vi "Preview Pop Up.vi"(6 "Local Data":T1, 7 "UI References":T8, 8 "error in (no error)":errorcluster, 9 "Side":enum16{"Left", "Right"}(ring)=enum."Right", 10 "Coords":T9) -> (0 "error out":errorcluster, 4 "Local Data Out":T1)   [LabVIEW 2024]
uses:
  <vilib>/Utility/miscctls.llb/LVPoint32TypeDef.ctl
  Controls/RVHR - UI Refs.ctl
  Controls/Test Cluster.ctl
  Controls/Excluded Information.ctl
  Controls/Language.ctl
  Controls/Device_Type.ctl
  <vilib>/Utility/miscctls.llb/LVRectTypeDef.ctl
  <vilib>/Utility/miscctls.llb/LVBoundsTypeDef.ctl
  Controls/RVHR - Local Data.ctl
panel:
  out "element":u32
  out "Zoom Picture":picture
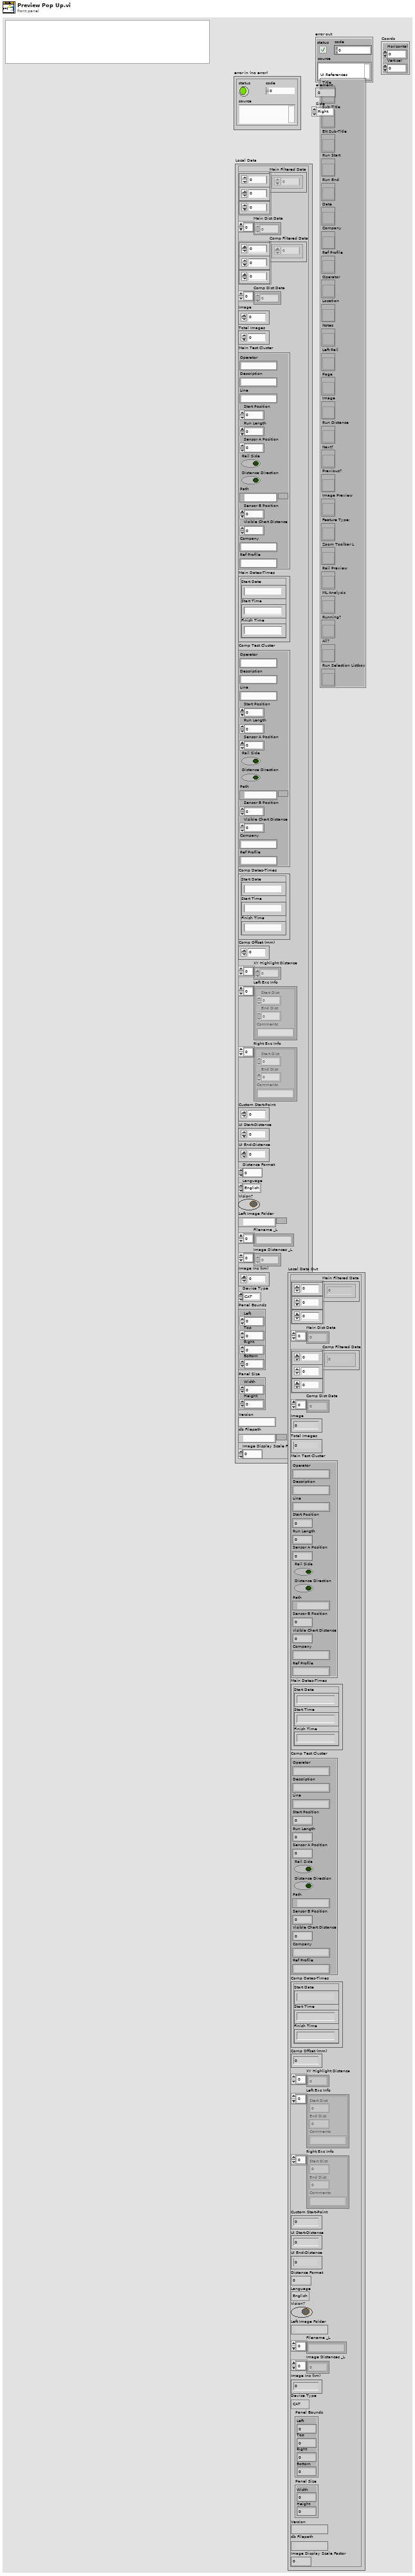
[diagram p1: front panel]
types:
  T1 = typedef "RVHR - Local Data.ctl" = cluster{"Main Filtered Data":dbl[][][], "Main Dist Data":dbl[], "Comp Filtered Data":dbl[][][], "Comp Dist Data":dbl[], "Image":u16, "Total Images":u16, "Main Test Cluster":T2, "Main Dates-Times":cluster{"Start Date":string, "Start Time":string, "Finish Time":string}, "Comp Test Cluster":T2, "Comp Dates-Times":cluster{"Start Date":string, "Start Time":string, "Finish Time":string}, "Comp Offset (mm)":i64, "XY Highlight Distance":dbl[], "Left Exc Info":T3[], "Right Exc Info":T3[], "Custom Start-Point":dbl, "UI Start-Distance":dbl, "UI End-Distance":dbl, "Distance Format":u8, "Language":T4, "Vision?":bool, "Left Image Folder":path, "Filename _L":string[], "Image Distances _L":dbl[], "Image Inc (km)":dbl, "Device Type":T5, "Panel Bounds":T6, "Panel Size":T7, "Version":string, "db Filepath":path, "Image Display Scale Factor":dbl}
  T2 = typedef "Test Cluster.ctl" = cluster{"Operator":string, "Description":string, "Line":string, "Start Position":dbl, "Run Length":dbl, "Sensor A Position":dbl, "Rail Side":bool, "Distance Direction":bool, "Path":path, "Sensor B Position":dbl, "Visible Chart Distance":dbl, "Company":string, "Ref Profile":string}
  T3 = typedef "Excluded Information.ctl" = cluster{"Start Dist":dbl, "End Dist":dbl, "Comments":string}
  T4 = typedef "Language.ctl" = enum16{"English", "Chinese", "German"}
  T5 = typedef "Device_Type.ctl" = enum16{"CAT", "Bi-CAT", "YRCA", "RCA", "RV-HR", "TV-HR"}
  T6 = typedef "LVRectTypeDef.ctl" = cluster{"Left":i16, "Top":i16, "Right":i16, "Bottom":i16}
  T7 = typedef "LVBoundsTypeDef.ctl" = cluster{"Width":u32, "Height":u32}
  T8 = typedef "RVHR - UI Refs.ctl" = cluster{"Title":refnum<vi>, "Sub-Title":refnum<vi>, "EN Sub-Title":refnum<vi>, "Run Start":refnum<vi>, "Run End":refnum<vi>, "Date":refnum<vi>, "Company":refnum<vi>, "Ref Profile":refnum<vi>, "Operator":refnum<vi>, "Location":refnum<vi>, "Notes":refnum<vi>, "Left Rail":refnum<vi>, "Page":refnum<vi>, "Image":refnum<vi>, "Run Distance":refnum<vi>, "Next?":refnum<vi>, "Previous?":refnum<vi>, "Image Preview":refnum<vi>, "Feature Type:":refnum<vi>, "Zoom Toolbar L":refnum<vi>, "Rail Preview":refnum<vi>, "ML Analysis":refnum<vi>, "Running?":refnum<vi>, "All?":refnum<vi>, "Run Selection Listbox":refnum<vi>}
  T9 = typedef "LVPoint32TypeDef.ctl" = cluster{"Horizontal":i32, "Vertical":i32}
  T10 = enum32{"Invalid", "Standard", "Closed", "Hidden", "Minimized", "Maximized"}
  T11 = typedef "LVMouseTypeDef.ctl" = cluster{"Mouse Position":cluster{"X":i32, "Y":i32}, "Mouse Modifiers":cluster{"Button Down":bool, "Shift Mod":bool, "Menu Mod":bool, "Option Mod":bool}}
  T12 = typedef "imagedata.ctl" = cluster{"image type":i32, "image depth":i32, "image":u8[], "mask":u8[], "colors":u32[], "Rectangle":cluster{"left":i16, "top":i16, "right":i16, "bottom":i16}}
  T13 = cluster{"left":i16, "top":i16, "right":i16, "bottom":i16}
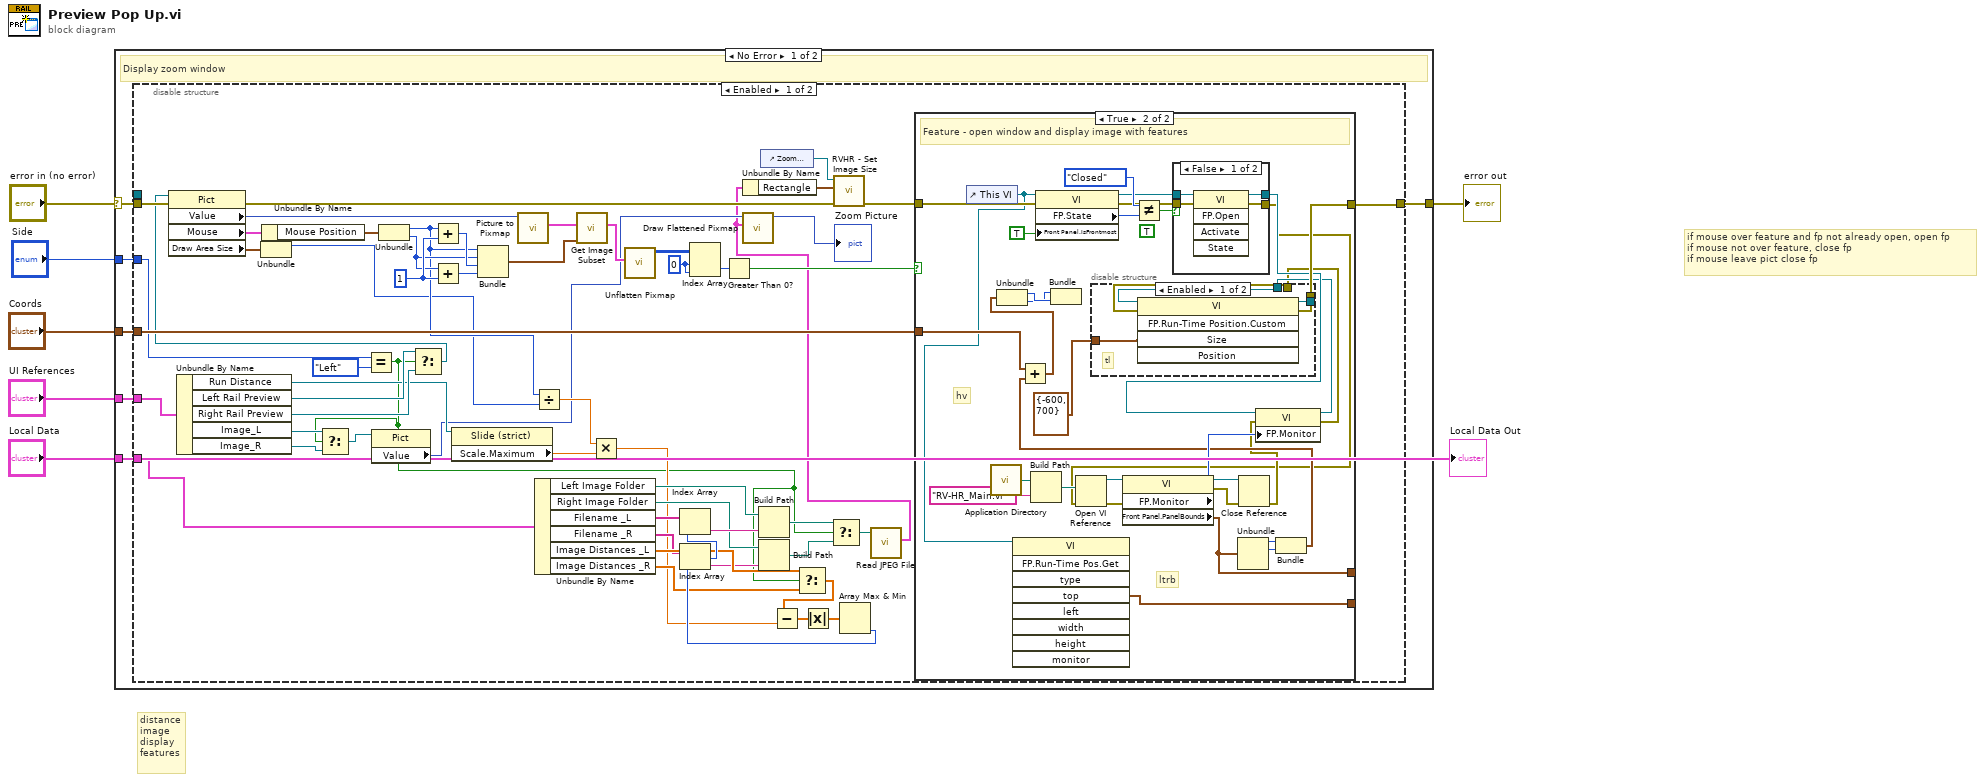
[diagram p0: block diagram]
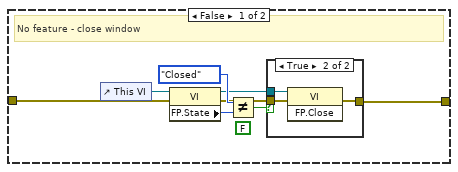
[diagram p2: hidden frame]
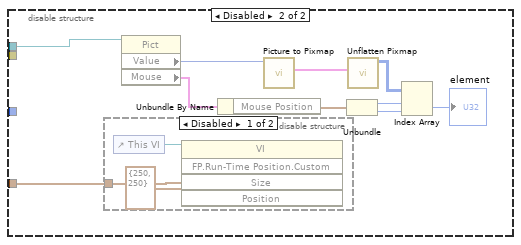
[diagram p6: hidden frame]
diagram:
  # "distance\nimage\ndisplay\nfeatures"
  # "if mouse over feature and fp not already open, open fp\nif mouse not over feature, close fp\nif mouse leave pict close fp"
  n1 = case shown="No Error" "error in (no error)" {
    selector: "error in (no error)" -> [w12 w138]
    tunnel: [w11 w138] -> w5
    tunnel: "Coords" -> [w10 _]
    tunnel: "UI References" -> [w9 _]
    tunnel: "Side" -> [w8 _]
    tunnel: "Local Data" -> [w7 _]
    frame No Error {
      # "Display zoom window"
      n2 = disable-structure shown="Enabled" {
        disable-tunnel: w12 -> [w67 _]
        disable-tunnel: _ -> [_ w133]
        disable-tunnel: [w49 _] -> w11
        disable-tunnel: w10 -> [w52 w134]
        disable-tunnel: w9 -> [w48 _]
        disable-tunnel: w8 -> [w47 _]
        disable-tunnel: w7 -> [w22 _]
        frame Enabled {
          w54 = 0 ("index (row)")
          w58 = 1 ("y")
          n3 = Unbundle By Name(w48) -> ("Run Distance"=w42:refnum<vi>, "Left Rail Preview"=w44:refnum<vi>, "Right Rail Preview"=w45:refnum<vi>, "Image_L"=w19:refnum<vi>, "Image_R"=w18:refnum<vi>)
          n4 = Equal?(x=w47, y=enum16{"Left", "Right"}."Left" ("Side")) -> (x = y?=w17:bool)
          n5 = Select(t=w19, s=w17, f=w18) -> (s? t:f=w16:refnum<vi>)
          n6 = property class="Pict"(reference=w16) -> ("Value"=w15:picture)  [unwired: 1 in, 2 out]
          n7 = Select(t=w44, s=w17, f=w45) -> (s? t:f=w43:refnum<vi>)
          n8 = property class="Pict"(reference=w43, error in=w67) -> (error out=w61:errorcluster, "Value"=w69:picture, "Mouse"=w60:T11, "Draw Area Size"=w41:T7)  [unwired: 1 out]
          n9 = Unbundle(w41) -> ("Width"=w37:u32)  [unwired: 1 out]
          n10 = Unbundle By Name(w60) -> ("Mouse Position"=w59:cluster{"X":i32, "Y":i32})
          n11 = Unbundle(w59) -> ("X"=w38:i32, "Y"=w56:i32)
          n12 = Add(x=w38, y=w58) -> (x+y=w65:i32)
          n13 = Add(x=w56, y=w58) -> (x+y=w64:i32)
          n14 = property class="Slide (strict)"(reference=w42) -> ("Scale.Maximum"=w40:dbl)  [unwired: 1 in, 2 out]
          n15 = Bundle("X"=w38, "Y"=w56, w65, w64) -> (w66:cluster{"X":i32, "Y":i32, i32, i32})  [unwired: 1 in]
          n16 = call <vilib>:"Picture to Pixmap.vi"("picture"=w69) -> ("image data"=w63:T12)  [unwired: 9 in, 1 out]
          n17 = Divide(x=w38, y=w37) -> (x/y=w39:dbl)
          n18 = Unbundle By Name(w22) -> ("Left Image Folder"=w23:path, "Right Image Folder"=w24:path, "Filename _L"=w25:string[], "Filename _R"=w26:string[], "Image Distances _L"=w34:dbl[], "Image Distances _R"=w35:dbl[])
          n19 = call <vilib>:"Get Image Subset.vi"("subset rect"=w66, "image data"=w63) -> ("image subset"=w57:T12)  [unwired: 4 in, 1 out]
          n20 = Multiply(x=w39, y=w40) -> (x*y=w21:dbl)
          n21 = call <vilib>:"Unflatten Pixmap.vi"("image data"=w57) -> ("24-bit pixmap"=w55:u32[][])  [unwired: 4 in, 6 out]
          n22 = Index Array(array=w55, index (row)=w54, index (col)=w54) -> (element=w53:u32)
          n23 = Greater Than 0?(x=w53) -> (x > 0?=w51:bool)
          n24 = control-ref of="Zoom Picture"() -> (w13:refnum<vi>)
          n25 = Select(t=w34, s=w17, f=w35) -> (s? t:f=w33:dbl[])
          n26 = Subtract(x=w33, y=w21) -> (x-y=w32:dbl[])
          n27 = Absolute Value(x=w32) -> (abs(x)=w31:dbl[])
          n28 = Array Max & Min(array=w31) -> (min index (indices)=w36:i32)  [unwired: 3 out]
          n29 = Index Array(array=w25, index=w36) -> (element=w27:string)
          n30 = Index Array(array=w26, index=w36) -> (element=w28:string)
          n31 = Build Path(base path=w23, name or relative path=w27) -> (appended path=w29:path)
          n32 = Build Path(base path=w24, name or relative path=w28) -> (appended path=w30:path)
          n33 = Select(t=w29, s=w17, f=w30) -> (s? t:f=w20:path)
          n34 = call <vilib>:"Read JPEG File.vi"("path to JPEG file"=w20) -> ("image data"=w14:T12)  [unwired: 8 in, 2 out]
          n35 = Unbundle By Name(w14) -> ("Rectangle"=w62:T13)
          n36 = call <vilib>:"Draw Flattened Pixmap.vi"("image data"=w14, "picture"=w15) -> ("new picture"=→"Zoom Picture":picture)  [unwired: 7 in]
          n37 = call "RVHR - Set Image Size.vi"("error in (no error)"=w61, "Rectangle"=w62, "Image_L"=w13) -> ("error out"=w50:errorcluster)  [unwired: 8 in]
          n38 = case shown="True" w51 {
            tunnel: w52 -> [_ w90]
            tunnel: w50 -> [w76 w113]
            tunnel: [w71 w108] -> w49
            tunnel: [_ w98] -> _
            tunnel: [_ w83] -> _
            frame False {
              (unwired) FALSE
              # "No feature - close window"
              n39 = control-ref of="This VI"() -> (w77:refnum<vi>)
              n40 = property class="VI"(reference=w77, error in=w76) -> (reference out=w72:refnum<vi>, error out=w73:errorcluster, "FP.State"=w75:T10)
              n41 = Not Equal?(x=T10."Closed" ("Front Panel Window:State"), y=w75) -> (x != y?=w70:bool)
              n42 = case shown="True" w70 {
                tunnel: w73 -> [w78 w80]
                tunnel: w72 -> [_ w81]
                tunnel: [w78 w79] -> w71
                frame False {
                }
                frame True {
                  n43 = invoke class="VI" method="FP.Close"(reference=w81, error in=w80) -> (error out=w79:errorcluster)  [unwired: 1 in, 2 out]
                }
              }
            }
            frame True {
              (unwired) TRUE
              # "hv"
              # "ltrb"
              # "Feature - open window and display image with features"
              n44 = control-ref of="This VI"() -> (w82:refnum<vi>)
              n45 = call <vilib>:"Application Directory.vi"() -> ("Application Directory"=w107:path)
              n46 = invoke class="VI" method="FP.Run-Time Pos.Get"(reference=w82) -> ("top"=w83:cluster{"Top":i16, "Left":i16})  [unwired: 8 in, 8 out]
              n47 = Build Path(base path=w107, name or relative path="RV-HR_Main.vi") -> (appended path=w105:path)
              n48 = property class="VI"(reference=w82, error in=w113, "Front Panel.IsFrontmost"=TRUE ("Front Panel Window:Is Frontmost")) -> (reference out=w109:refnum<vi>, error out=w110:errorcluster, "FP.State"=w112:T10)
              n49 = Not Equal?(x=T10."Closed" ("Front Panel Window:State"), y=w112) -> (x != y?=w94:bool)
              n50 = case shown="False" w94 {
                tunnel: w110 -> [w121 w124]
                tunnel: w109 -> [w122 w123]
                tunnel: [w120 w124] -> w85
                tunnel: [w119 w123] -> w103
                frame False {
                  n51 = invoke class="VI" method="FP.Open"(reference=w122, error in=w121) -> (reference out=w119:refnum<vi>, error out=w120:errorcluster)  [unwired: 3 in, 3 out]
                }
                frame True {
                }
              }
              n52 = Open VI Reference(vi path=w105, error in (no error)=w85) -> (vi reference=w104:refnum<vi>, error out=w102:errorcluster)  [unwired: 4 in]
              n53 = property class="VI"(reference=w104, error in=w102) -> (reference out=w100:refnum<vi>, error out=w101:errorcluster, "FP.Monitor"=w99:u16, "Front Panel.PanelBounds"=w98:T6)
              n54 = Unbundle(w98) -> ("Left"=w97:i16, "Top"=w96:i16)  [unwired: 2 out]
              n55 = Close Reference(reference=w100, error in (no error)=w101) -> (error out=w86:errorcluster)
              n56 = property class="VI"(reference=w103, error in=w86, "FP.Monitor"=w99) -> (reference out=w88:refnum<vi>, error out=w87:errorcluster)
              n57 = disable-structure shown="Enabled" {
                disable-tunnel: w88 -> [w116 _]
                disable-tunnel: w87 -> [w118 _]
                disable-tunnel: [w117 _] -> w108
                disable-tunnel: [w115 _] -> _
                disable-tunnel: cluster{"Vertical":i32, "Horizontal":i32} {"Vertical"=-600, "Horizontal"=700} -> [w114 _]
                frame Enabled {
                  # "tl"
                  n58 = invoke class="VI" method="FP.Run-Time Position.Custom"(reference=w116, error in=w118, "Size"=w114) -> (reference out=w115:refnum<vi>, error out=w117:errorcluster)  [unwired: 2 in, 3 out]
                }
                frame Disabled {
                }
              }
              n59 = Bundle("Left"=w97, "Top"=w96) -> (w95:cluster{"Left":i16, "Top":i16})  [unwired: 1 in]
              n60 = Add(x=w90, y=w95) -> (x+y=w89:T9)
              n61 = Unbundle(w89) -> ("Horizontal"=w92:i32, "Vertical"=w91:i32)
              n62 = Bundle("Vertical"=w91, "Horizontal"=w92) -> ()  [unwired: 1 in, 1 out]
            }
          }
        }
        frame Disabled {
          n63 = disable-structure shown="Disabled" {
            disable-tunnel: w134 -> [w136 _]
            frame Disabled {
              n64 = control-ref of="This VI"() -> (w137:refnum<vi>)
              n65 = invoke class="VI" method="FP.Run-Time Position.Custom"(reference=w137, "Size"=w136, "Position"=cluster{"Height":i16, "Width":i16} {"Height"=250, "Width"=250} ("Size")) -> ()  [unwired: 2 in, 5 out]
            }
            frame Enabled {
            }
          }
          n66 = property class="Pict"(reference=w133) -> ("Value"=w132:picture, "Mouse"=w131:T11)  [unwired: 1 in, 2 out]
          n67 = Unbundle By Name(w131) -> ("Mouse Position"=w130:cluster{"X":i32, "Y":i32})
          n68 = call <vilib>:"Picture to Pixmap.vi"("picture"=w132) -> ("image data"=w127:T12)  [unwired: 9 in, 1 out]
          n69 = Unbundle(w130) -> ("X"=w129:i32, "Y"=w128:i32)
          n70 = call <vilib>:"Unflatten Pixmap.vi"("image data"=w127) -> ("24-bit pixmap"=w125:u32[][])  [unwired: 4 in, 6 out]
          n71 = Index Array(array=w125, index (row)=w129, index (col)=w128) -> (element=→"element":u32)
        }
      }
    }
    frame Error {
    }
  }
  "error out" <- w5
  "Local Data Out" <- "Local Data"
